vi "Initialize.vi"(7 "Channel Name":string="ActualValue.ch%d.AV", 8 "error in":errorcluster, 9 "Number of Channels":u32=1, 10 "Instance Name":string, 11 "Nominal Value in":refnum<class "Nominal Value.lvclass">) -> (0 "error out":errorcluster, 3 "Nominal Value out":refnum<class "Nominal Value.lvclass">)   [LabVIEW 2023, in "Nominal Value.lvclass"]
uses:
  Nominal Value.lvclass
  Nominal Value.lvclass/Nominal Value.ctl
  <vilib>/ADAS Replay HIL/Channels/Tag Wrapper/Tag Wrapper.lvlib
  Utilities/Utilities.lvlib
  <vilib>/ADAS Replay HIL/Channels/Tag Wrapper/Polymorphic/Open Producer Tag (Double).vi
  <vilib>/ADAS Replay HIL/Channels/Tag Wrapper/Polymorphic/Set Default Value (Double).vi
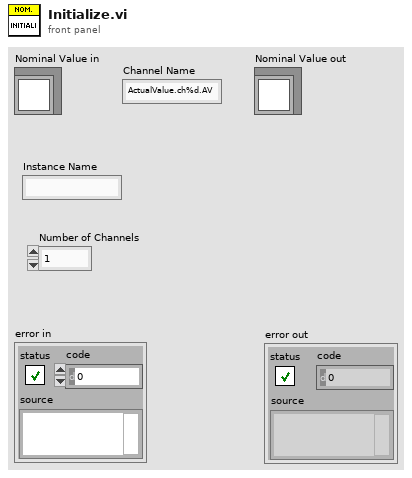
[diagram p1: front panel]
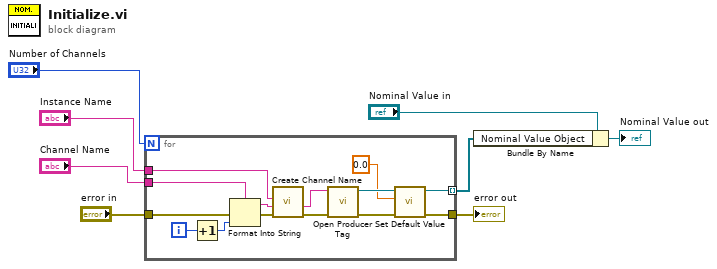
[diagram p0: block diagram]
diagram:
  n1 = for {
    N: "Number of Channels" -> [_]
    tunnel: [w15] -> w4 mode=indexing
    tunnel: [w14] -> w5
    tunnel: "Channel Name" -> [w22]
    tunnel: "Instance Name" -> [w12]
    tunnel: "error in" -> [w19]
    i -> [w21]
    n2 = Increment(x=w21) -> (x+1=w20:i32)
    n3 = Format Into String(format string=w22, error in=w19, w20) -> (resulting string=w13:string, error out=w10:errorcluster)  [unwired: 1 in]
    n4 = call "Create Channel Name.vi"("error in"=w10, "Channel Name"=w13, "Plugin Name"=w12) -> ("error out"=w9:errorcluster, "Data Channel Name"=w11:string)  [unwired: 7 in]
    n5 = call-poly <vilib>:"Open Producer Tag.vi"("error in"=w9, "Channel Name"=w11) -> ("error out"=w18:errorcluster, "ADAS HIL Channel"=w17:refnum<k21>)  [unwired: 8 in]
    n6 = call-poly <vilib>:"Set Default Value.vi"("error in"=w18, "Default Value"=0.0, "ADAS HIL Channel in"=w17) -> ("error out"=w14:errorcluster, "ADAS HIL Channel out"=w15:refnum<k21>)  [unwired: 7 in]
  }
  "error out" <- w5
  n7 = Bundle By Name(cluster="Nominal Value in", "Nominal Value Object"=w4) -> (→"Nominal Value out":refnum<class "Nominal Value.lvclass">)
